vi "enable_Output_PSG.vi"(8 "error in (no error)":errorcluster, 10 "Enable RF Output (F:Disable)":bool, 11 "VISA resource name":refnum<visa-resource-name>) -> (0 "error out":errorcluster, 3 "VISA resource name out":refnum<visa-resource-name>)   [LabVIEW 2011]
doc: "Configures RF output, modulation state, blanking, and RPP circuit of the signal generator."
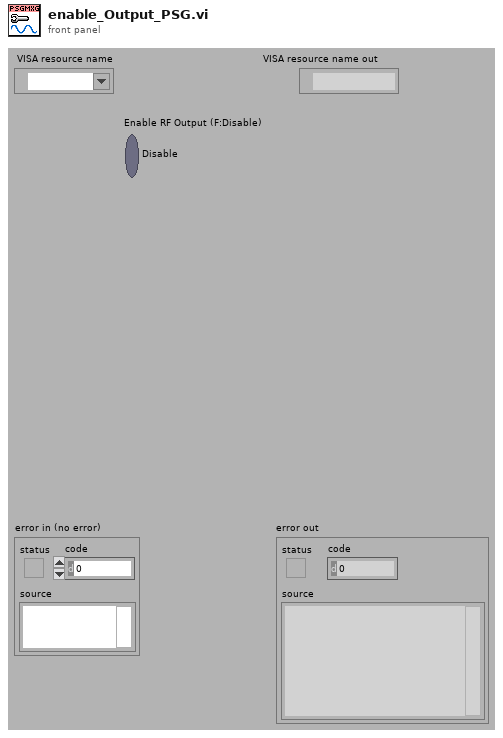
[diagram p1: front panel]
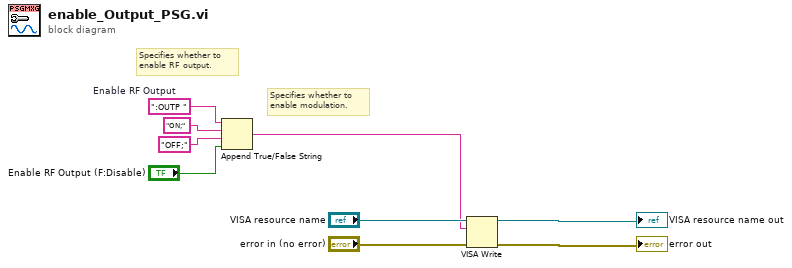
[diagram p0: block diagram]
diagram:
  w9 = ":OUTP "  # Enable RF Output
  # "Specifies whether to\nenable modulation."
  # "Specifies whether to\nenable RF output."
  n1 = Append True/False String(1:"Enable RF Output (F:Disable)", 2:"OFF;" ("false string"), 3:"ON;" ("true string"), 4:w9) -> (0:w3:string)
  n2 = VISA Write(VISA resource name="VISA resource name", write buffer=w3, error in (no error)="error in (no error)") -> (VISA resource name out=→"VISA resource name out":refnum<visa-resource-name>, error out=→"error out":errorcluster)  [unwired: 1 out]
